vi "Check_connection.vi"(2 "error in (no error)":errorcluster) -> (8 "Internet Connected?":bool, 9 "error out":errorcluster)   [LabVIEW 2016]
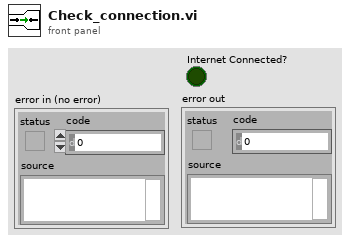
[diagram p1: front panel]
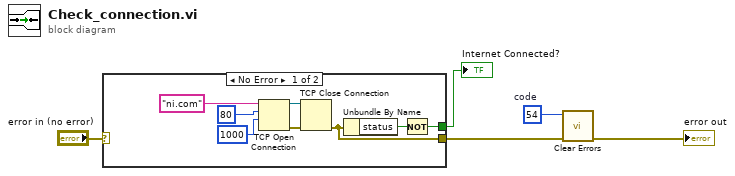
[diagram p0: block diagram]
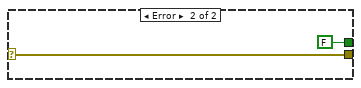
[diagram p2: hidden frame]
diagram:
  w1 = 54  # code
  n1 = case shown="No Error" "error in (no error)" {
    selector: "error in (no error)" -> [_ w14]
    tunnel: [w8 FALSE] -> w4
    tunnel: [w7 w14] -> w2
    frame No Error {
      n2 = TCP Open Connection(address="ni.com", remote port or service name=u16 80, timeout ms (60000)=1000) -> (connection ID=w12:refnum<k5>, error out=w13:errorcluster)  [unwired: 2 in]
      n3 = TCP Close Connection(connection ID=w12, error in (no error)=w13) -> (error out=w7:errorcluster)  [unwired: 1 in, 1 out]
      n4 = Unbundle By Name(w7) -> ("status"=w9:bool)
      n5 = Not(x=w9) -> (.not. x?=w8:bool)
    }
    frame Error {
    }
  }
  "Internet Connected?" <- w4
  n6 = call <vilib>:"Clear Errors.vi"("error in (no error)"=w2, "specific error code to clear (0: all)"=w1) -> ("error out"=→"error out":errorcluster)  [unwired: 4 in, 1 out]
